vi "Test Triangle Class.vi"(8 "error in (no error)":errorcluster, 11 "TestCase in":refnum<class "Test FGEN.lvclass">) -> (0 "error out":errorcluster, 3 "TestCase out":refnum<class "Test FGEN.lvclass">)   [LabVIEW 2020, in "Test FGEN.lvclass"]
uses:
  Test FGEN.lvclass
  Libraries/FGen/Generador/Generador.lvclass
  <vilib>/addons/_JKI Toolkits/VI Tester/TestCase.llb/TestCase.lvclass
  C:/Program Files (x86)/National Instruments/LabVIEW 2020/vi.lib/addons/_JKI Toolkits/VI Tester/TestCase.llb/TestCase.lvclass
panel:
  out "Triangle Constant":waveform(dbl)
  out "Waveform":waveform(dbl)
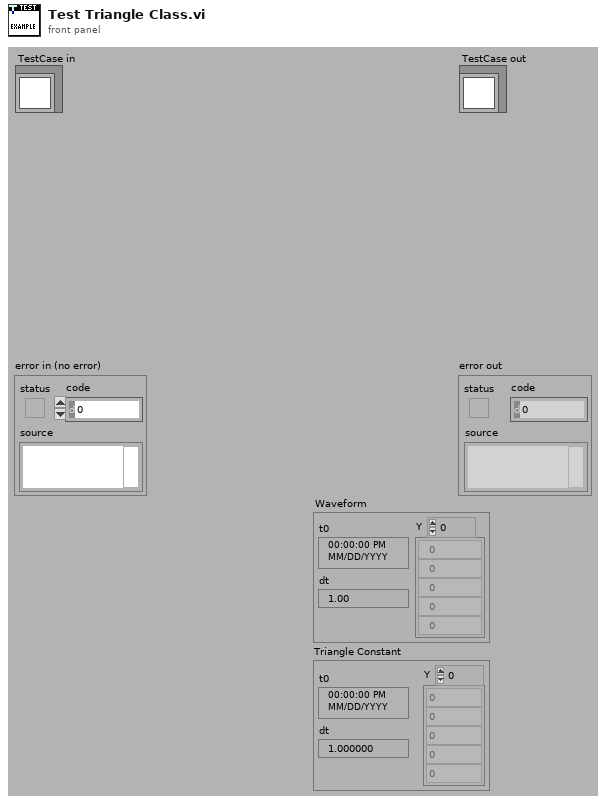
[diagram p1: front panel]
types:
  T1 = enum16{"Sine Wave", "Triangle Wave", "Square Wave", "Sawtooth Wave"}
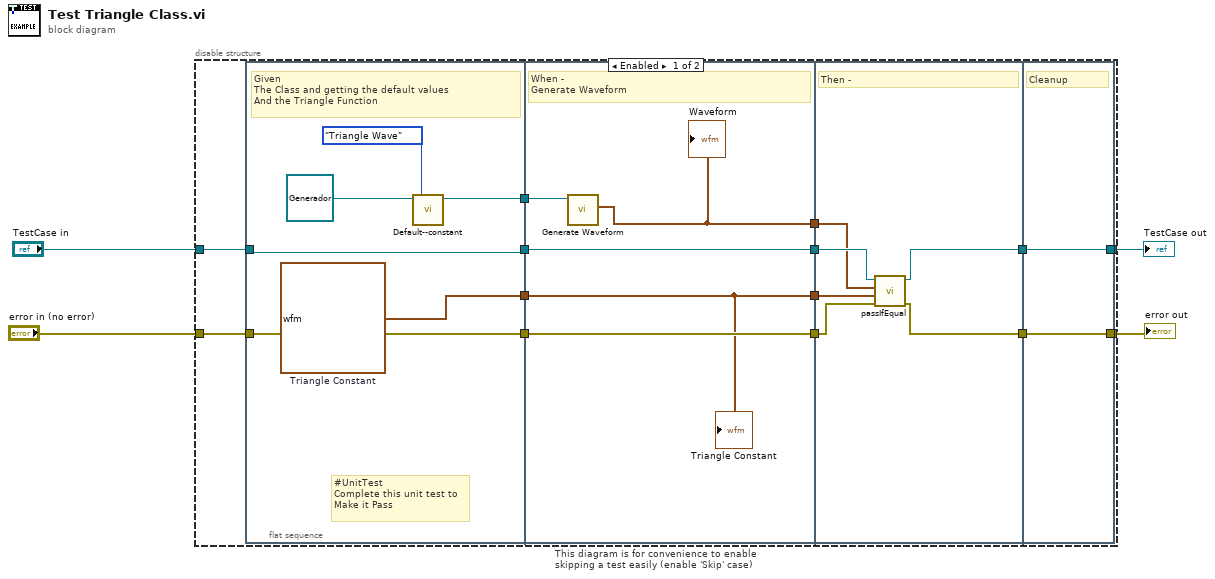
[diagram p0: block diagram]
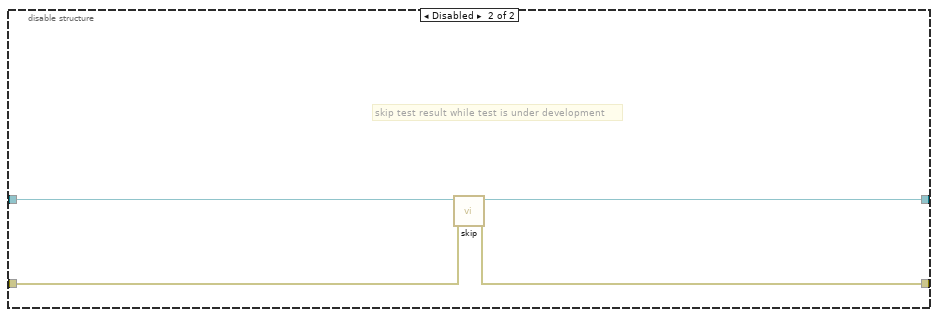
[diagram p2: hidden frame]
diagram:
  n1 = disable-structure "This diagram is for convenience to enable skipping a test easily (enable 'Skip' case)" shown="Enabled" {
    disable-tunnel: "TestCase in" -> [w14 w41]
    disable-tunnel: [w12 w39] -> w1
    disable-tunnel: [w13 w40] -> w3
    disable-tunnel: "error in (no error)" -> [w11 w38]
    frame Enabled {
      n2 = flat-sequence {
        tunnel: w14 -> [w24]
        tunnel: [w24] -> w18
        tunnel: w11 -> [w23]
        tunnel: [w23] -> w9
        tunnel: [w22] -> w7
        tunnel: [w21] -> w6
        tunnel: [w29] -> w17
        tunnel: w18 -> [w29]
        tunnel: [w28] -> w10
        tunnel: w9 -> [w28]
        tunnel: [w27] -> w8
        tunnel: w7 -> [w27]
        tunnel: w6 -> [w26]
        tunnel: [w25] -> w5
        tunnel: [w34] -> w16
        tunnel: [w33] -> w15
        tunnel: w17 -> [w35]
        tunnel: w10 -> [w32]
        tunnel: w8 -> [w31]
        tunnel: w5 -> [w30]
        tunnel: [w36] -> w13
        tunnel: [w37] -> w12
        tunnel: w16 -> [w37]
        tunnel: w15 -> [w36]
        frame #0 {
          w22 = waveform(dbl) {"t0"=timestamp(0 s since 1904-01-01), "dt"=0.001, "Y"=array[1000 elements]}  # Triangle Constant
          # "#UnitTest\nComplete this unit test to\nMake it Pass"
          # "Given\nThe Class and getting the default values\nAnd the Triangle Function"
          n3 = call-dynamic "Default--constant.vi"("signal type"=T1."Triangle Wave", "Generator in"=refnum<class "Generador.lvclass"> refnum ("FGen.lvlib:Generator")) -> ("Generator out"=w21:refnum<class "Generador.lvclass">)  [unwired: 8 in, 1 out]
        }
        frame #1 {
          # "When -\nGenerate Waveform"
          n4 = call "Generate Waveform.vi"("Generator in"=w26) -> ("Waveform"=w25:waveform(dbl))  [unwired: 8 in, 2 out]
          "Waveform" <- w25
          "Triangle Constant" <- w27
        }
        frame #2 {
          # "Then -"
          n5 = call-dynamic "passIfEqual.vi"("error in (no error)"=w32, "y"=w31, "x"=w30, "TestCase in"=w35) -> ("error out"=w33:errorcluster, "TestCase out"=w34:refnum<class "Test FGEN.lvclass">)  [unwired: 6 in]
        }
        frame #3 {
          # "Cleanup"
        }
      }
    }
    frame Disabled {
      # "skip test result while test is under development"
      n6 = call <vilib>:"skip.vi"("error in (no error)"=w38, "TestCase in"=w41) -> ("error out"=w40:errorcluster, "TestCase out"=w39:refnum<class "Test FGEN.lvclass">)  [unwired: 8 in]
    }
  }
  "error out" <- w3
  "TestCase out" <- w1
